vi "MU Calibration Get Optimized Nonius Track Offset Table Base Only.vi"(8 "error in (no error)":errorcluster, 11 "analyzeResult":T1) -> (0 "error out (no error)":errorcluster, 3 "optimizedNoniusTrackOffsetTableBaseOnly":cluster{"spoBase":i8, "spoN":i8[]})   [LabVIEW 2017, in "MU_3SL_interface.lvlib"]
uses:
  MU_3SL_interface.lvlib
  handles/CalibrationAnalyzeResultHandle.ctl
  lib/MU_3SL_interface.dll
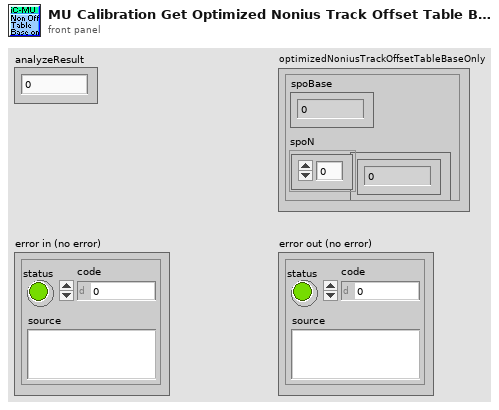
[diagram p1: front panel]
types:
  T1 = typedef "MU_3SL_interface.lvlib/CalibrationAnalyzeResultHandle.ctl" = u64
  T2 = cluster{"[0]":i8, "[1]":i8, "[2]":i8, "[3]":i8, "[4]":i8, "[5]":i8, "[6]":i8, "[7]":i8, "[8]":i8, "[9]":i8, "[10]":i8, "[11]":i8, "[12]":i8, "[13]":i8, "[14]":i8, "[15]":i8, "[16]":i8}
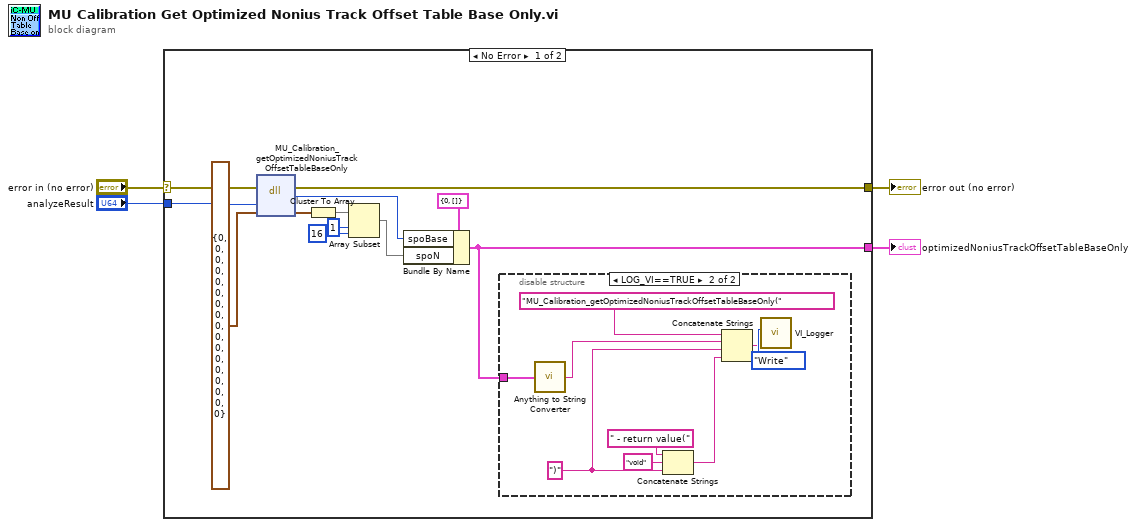
[diagram p0: block diagram]
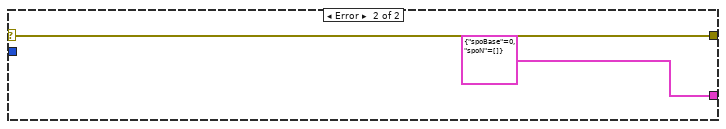
[diagram p3: hidden frame]
diagram:
  n1 = case shown="No Error" "error in (no error)" {
    selector: "error in (no error)" -> [w16 w27]
    tunnel: [w14 w27] -> w4
    tunnel: "analyzeResult" -> [w15 _]
    tunnel: [w8 cluster{"spoBase":i8, "spoN":i8[]} {"spoBase"=0, "spoN"=[]} ("optimizedNoniusTrackOffsetTable")] -> w1
    frame No Error {
      n2 = dll-call lib="C:/Users/bes/AppData/Roaming/work/mu_9so/icsubmodules/soft_mu_3sl_master/lv_interface/lib/MU_3SL_interface**.*" fn="MU_Calibration_getOptimizedNoniusTrackOffsetTableBaseOnly"(error in=w16, "analyzeResult"=w15, "optimizedNoniusTrackOffsetTable"=T2 {"[0]"=0, "[1]"=0, "[2]"=0, "[3]"=0, "[4]"=0, "[5]"=0, "[6]"=0, "[7]"=0, "[8]"=0, "[9]"=0, "[10]"=0, "[11]"=0, "[12]"=0, "[13]"=0, "[14]"=0, "[15]"=0, "[16]"=0} ("cluster")) -> (error out=w14:errorcluster, "optimizedNoniusTrackOffsetBaseOnly"=w7:i8, "optimizedNoniusTrackOffsetTable"=w5:T2)  [unwired: 3 in, 1 out]
      n3 = Cluster To Array(cluster=w5) -> (array=w11:i8[])
      n4 = Array Subset(array=w11, index=1, length=16) -> (w10:i8[])
      n5 = Bundle By Name(cluster=cluster{"spoBase":i8, "spoN":i8[]} {"spoBase"=0, "spoN"=[]} ("optimizedNoniusTrackOffsetTable"), "spoBase"=w7, "spoN"=w10) -> (w8:cluster{"spoBase":i8, "spoN":i8[]})
      n6 = disable-structure shown="LOG_VI==TRUE" {
        disable-tunnel: w8 -> [_ w20]
        frame condition #0 {
        }
        frame condition #1 (active) {
          w19 = ")" ("string")
          n7 = call "Anything to String Converter.vi"("anything"=w20) -> ("String"=w18:string)
          n8 = Concatenate Strings(" - return value(" ("string"), "void" ("string"), w19) -> (w17:string)
          n9 = Concatenate Strings("MU_Calibration_getOptimizedNoniusTrackOffsetTableBaseOnly(" ("Info in"), w18, w19, w17) -> (w23:string)
          n10 = call "VI_Logger.vi"("Action (Read)"=enum16{"Write", "Read"}."Write", "Info in"=w23) -> ()  [unwired: 8 in, 2 out]
        }
      }
    }
    frame Error {
    }
  }
  "error out (no error)" <- w4
  "optimizedNoniusTrackOffsetTableBaseOnly" <- w1
